vi "Unpack for gRPC.vi"(8 "error in":errorcluster, 9 "configuration / results":enum16{"Configuration", "Results"}(ring), 10 "any":T1, 11 "measurement in":refnum<class "Continuous Counting Measurement.lvclass">) -> (0 "error out":errorcluster, 2 "data value":variant, 3 "measurement out":refnum<class "Continuous Counting Measurement.lvclass">)   [LabVIEW 2021, in "MeasurementServerTests.lvlib" / "Measurement Service Tests.lvlib" / "Continuous Counting Measurement.lvclass"]
uses:
  Continuous Counting Measurement.lvclass
  <vilib>/gRPC/LabVIEW gRPC Library/Shared/Any.ctl
  C:/Dev/github/ni/measurementlink-labview/Source/Runtime/Measurements/Measurement Plugin Service/Measurement Plugin Service.lvclass
  Measurement Configuration.ctl
  Measurement Results.ctl
  6d635c40-cdca-454d-9a33-8f7cce60832d.vi
  b8e90dfb-57be-4e27-95ee-452e096a7645.vi
  <vilib>/gRPC/LabVIEW gRPC Library/Server API/Translate Protobuf Error.vi
  <vilib>/AdvancedString/1D String Array to Delimited String.vi
  <vilib>/gRPC/LabVIEW gRPC Library/Server API/Server/Get Server DLL Path.vi
  Runtime/Measurements/Measurement Plugin Service/Measurement Plugin Service.lvclass
  <vilib>/gRPC/LabVIEW gRPC Library/grpc-lvsupport-release.lvlib
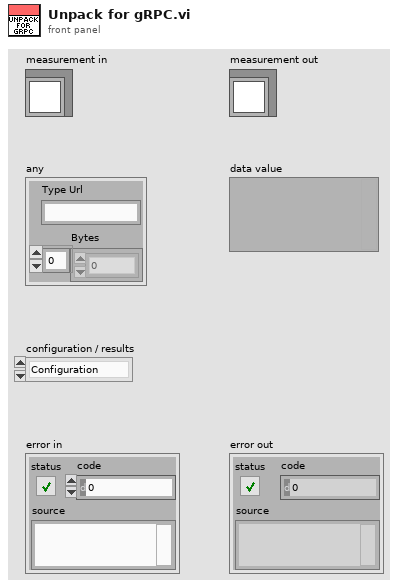
[diagram p1: front panel]
types:
  T1 = typedef "grpc-lvsupport-release.lvlib/Any.ctl" = cluster{"Type Url":string, "Bytes":u8[]}
  T2 = typedef "grpc-lvsupport-release.lvlib/grpcId.ctl" = u64
  T3 = typedef "MeasurementServerTests.lvlib/Measurement Service Tests.lvlib/Continuous Counting Measurement.lvclass/Measurement Configuration.ctl" = cluster{"ms update interval":u32}
  T4 = typedef "MeasurementServerTests.lvlib/Measurement Service Tests.lvlib/Continuous Counting Measurement.lvclass/Measurement Results.ctl" = cluster{"current count":i64}
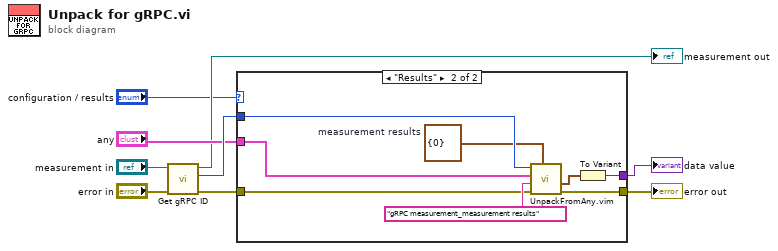
[diagram p0: block diagram]
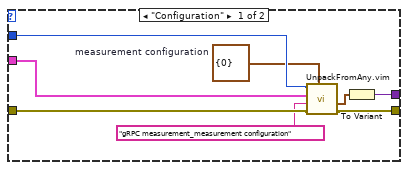
[diagram p2: hidden frame]
diagram:
  n1 = call "Get gRPC ID.vi"("error in"="error in", "measurement plugin service in"="measurement in") -> ("error out"=w9:errorcluster, "gRPC ID"=w8:T2, "measurement plugin service out"=→"measurement out":refnum<class "Continuous Counting Measurement.lvclass">)  [unwired: 7 in]
  n2 = case shown="\"Results\"" "configuration / results" {
    tunnel: w9 -> [w15 w20]
    tunnel: "any" -> [w11 w19]
    tunnel: w8 -> [w13 w22]
    tunnel: [w16 w23] -> w1
    tunnel: [w17 w25] -> w2
    frame "Configuration" {
      w10 = T3 {"ms update interval"=0}  # measurement configuration
      n3 = call "UnpackFromAny.vim"("Data Type"=w10, "error in"=w15, "Message Type"="gRPC measurement_measurement configuration", "Any"=w11, "gRPCid in"=w13) -> ("error out"=w16:errorcluster, "Unpacked Value"=w14:T3)  [unwired: 4 in, 1 out]
      n4 = To Variant(anything=w14) -> (Variant=w17:variant)
    }
    frame "Results" {
      w18 = T4 {"current count"=0}  # measurement results
      n5 = call "UnpackFromAny.vim"("Data Type"=w18, "error in"=w20, "Message Type"="gRPC measurement_measurement results", "Any"=w19, "gRPCid in"=w22) -> ("error out"=w23:errorcluster, "Unpacked Value"=w24:T4)  [unwired: 4 in, 1 out]
      n6 = To Variant(anything=w24) -> (Variant=w25:variant)
    }
  }
  "error out" <- w1
  "data value" <- w2
